vi "RH_Relays_Initialize.vi"(8 "error in":errorcluster, 11 "Relays Resource Name":refnum<k15>) -> (0 "error out":errorcluster, 3 "Relays Session Out":refnum<k15>)   [LabVIEW 2023, in "ResourceHandling.lvlib"]
doc: "Initialize NI PXI-2567 Relay boards"
uses:
  ResourceHandling.lvlib
  <instrlib>/niSwitch/niSwitch.llb/niSwitch Topologies.ctl
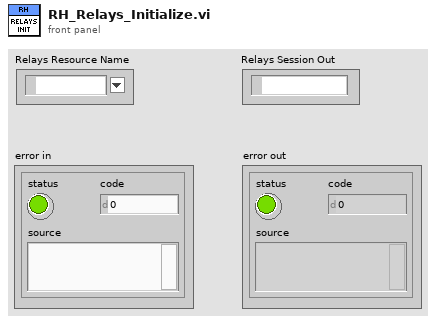
[diagram p1: front panel]
types:
  T1 = typedef "niSwitch Topologies.ctl" = string
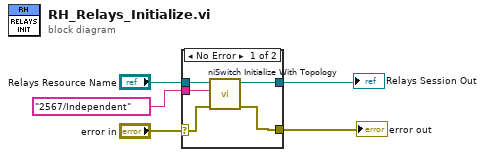
[diagram p0: block diagram]
diagram:
  n1 = case shown="No Error" "error in" {
    selector: "error in" -> [w6 w12]
    tunnel: "Relays Resource Name" -> [w10 w11]
    tunnel: T1 "2567/Independent" ("topology name") -> [w9 _]
    tunnel: [w8 w12] -> w3
    tunnel: [w7 w11] -> w4
    frame No Error {
      n2 = call <instrlib>:"niSwitch Initialize With Topology.vi"("error in (no error)"=w6, "topology name"=w9, "resource name"=w10) -> ("error out"=w8:errorcluster, "instrument handle out"=w7:refnum<k15>)  [unwired: 7 in]
    }
    frame Error {
    }
  }
  "error out" <- w3
  "Relays Session Out" <- w4
